vi "2 Cube Auto.vi"(11 "Right?":bool=TRUE) -> ()   [LabVIEW 2017]
uses:
  2 Cube Auto Type Def.ctl
  LabVIEW_is_Under_Control.lib/Util/Unpack Gamepad/D-Pad.ctl
  LabVIEW_is_Under_Control.lib/Util/Unpack Gamepad/Button Cluster.ctl
  Team Code/Robot Global Data.vi
panel:
  out "Enum":T1=enum."Finalizando"
  in  "Time to wait 4 (min 50ms)":dbl=50.0
  in  "DistanceFwd 4":dbl=100.0
  in  "Delay Fwd 4":i32=600
  in  "Time_Limit_fwd 4":dbl=2000.0 format="%#_13g"
  in  "Time_Limit_Turn 2":dbl=2000.0 format="%#_13g"
  in  "Turn 2":dbl=-110.0 format="%#_13g"
  in  "Delay Turn 2":i32=300
  in  "DistanceFwd 3":dbl=-60.0
  in  "Delay Fwd 3":i32=80
  in  "Time_Limit_fwd 3":dbl=2000.0 format="%#_13g"
  in  "Time to wait 3 (min 50ms)":dbl=50.0
  in  "DistanceFwd 2":dbl=55.0
  in  "Delay Fwd 2":i32=80
  in  "Time_Limit_fwd 2":dbl=1000.0 format="%#_13g"
  in  "Time to wait 2 (min 50ms)":dbl=50.0
  in  "Time_Limit_Turn":dbl=1500.0 format="%#_13g"
  in  "Turn":dbl=-30.0 format="%#_13g"
  in  "Delay Turn":i32=100
  in  "DistanceFwd":dbl=600.0
  in  "Delay Fwd":i32=300
  in  "Time_Limit_fwd":dbl=4800.0 format="%#_13g"
  in  "Time to wait (min 50ms)":dbl=100.0
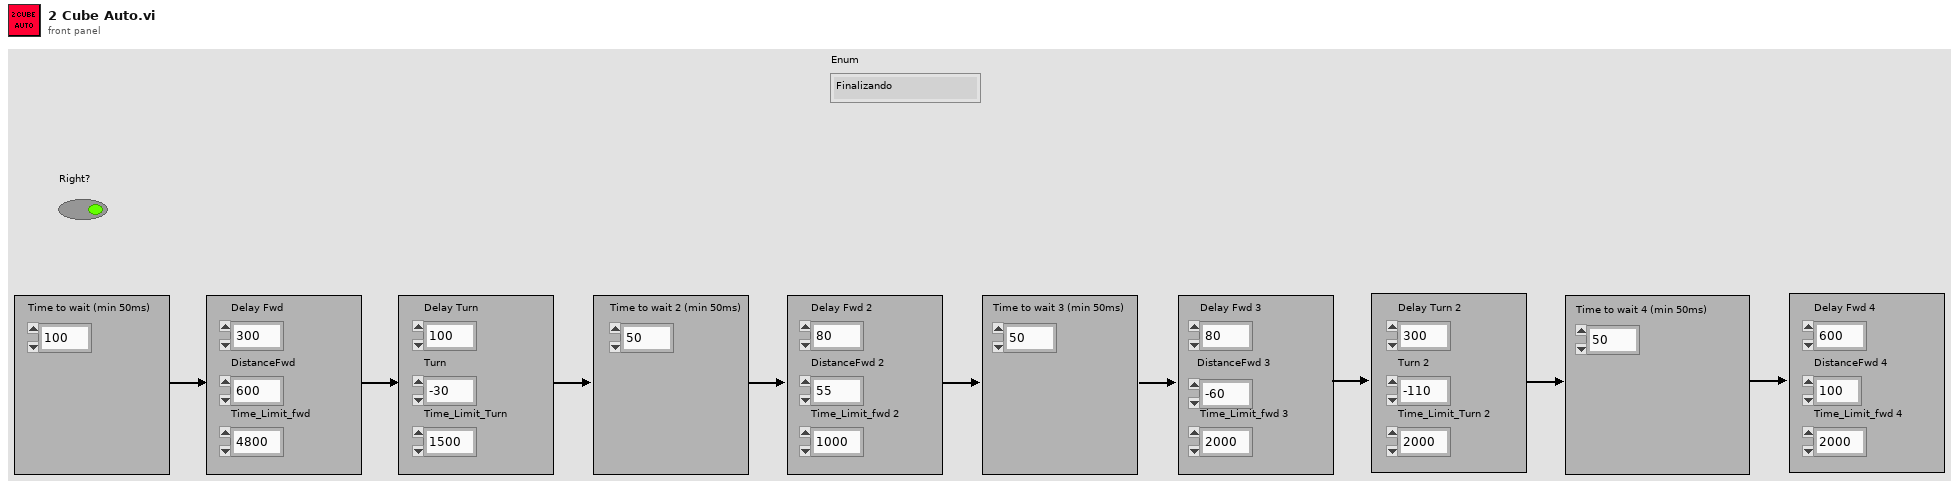
[diagram p1: front panel]
types:
  T1 = typedef "2 Cube Auto Type Def.ctl" = enum16{"Zerandosensor", "Andando", "Girando", "Zerandosensor2", "Andando2", "Score", "Zerandosensor3", "Andando3", "Girando2", "Zerandosensor4", "Andando4", "Elevator Up", "Score2", "Finalizando"}
  T2 = typedef "D-Pad.ctl" = cluster{"Top":bool, "Bottom":bool, "None":bool, "Right":bool, "Left":bool}
  T3 = cluster{"proportional gain (Kc)":dbl, "integral time (Ti, min)":dbl, "derivative time (Td, min)":dbl}
  T4 = typedef "Button Cluster.ctl" = cluster{"Buttons[0]":bool, "Buttons[1]":bool, "Buttons[2]":bool, "Buttons[3]":bool, "Buttons[4]":bool, "Buttons[5]":bool, "Buttons[6]":bool, "Buttons[7]":bool, "Buttons[8]":bool, "Buttons[9]":bool}
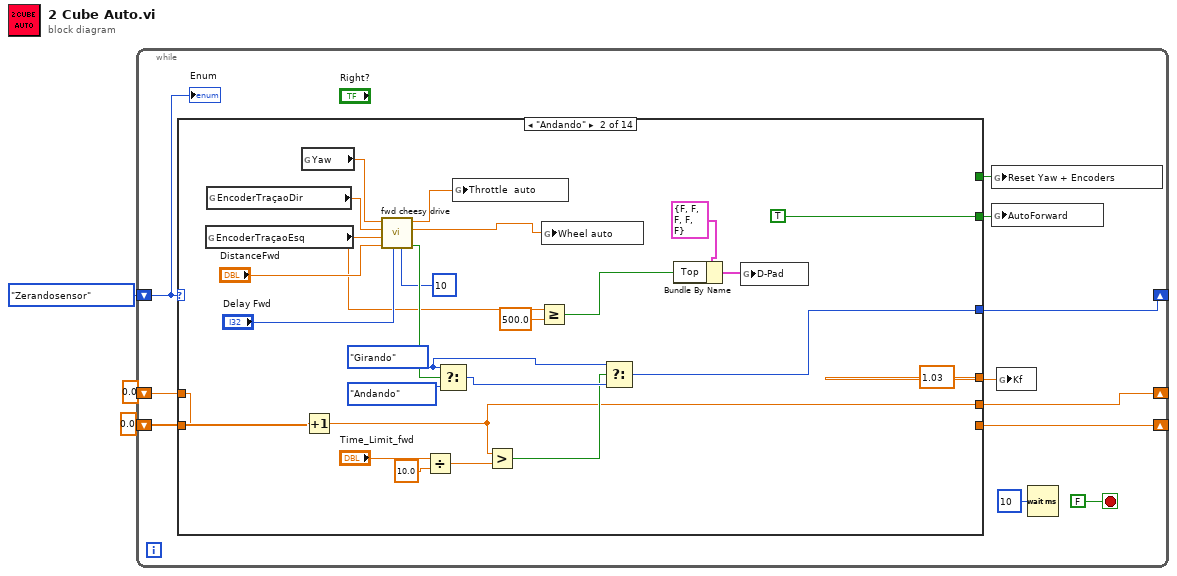
[diagram p0: block diagram]
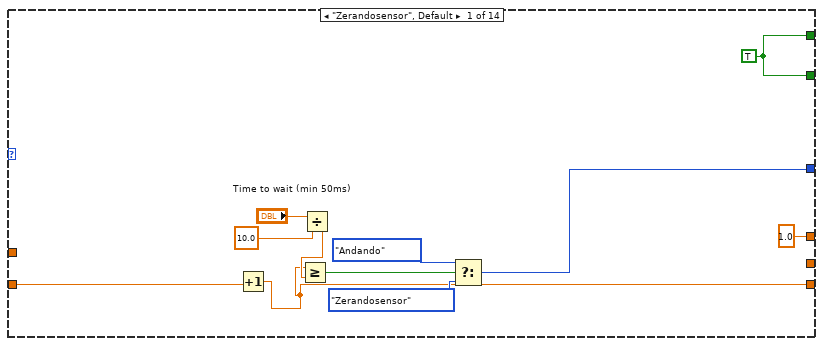
[diagram p2: hidden frame]
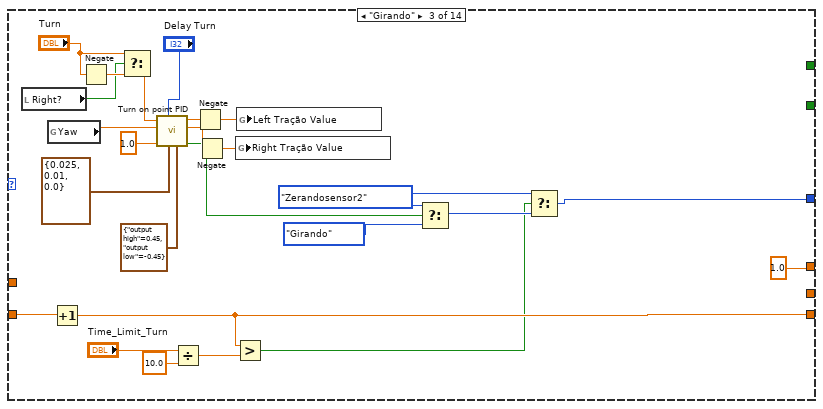
[diagram p3: hidden frame]
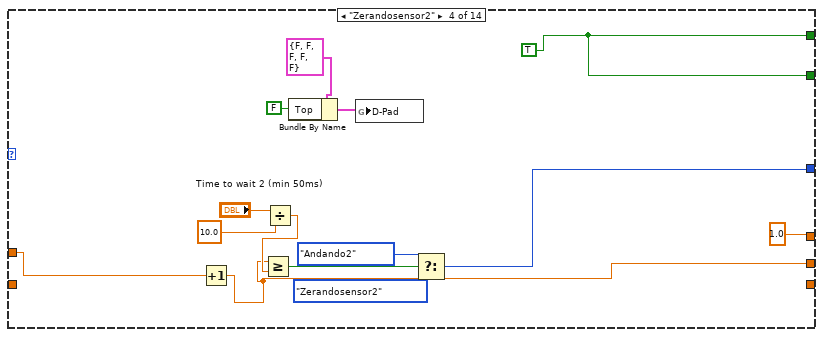
[diagram p4: hidden frame]
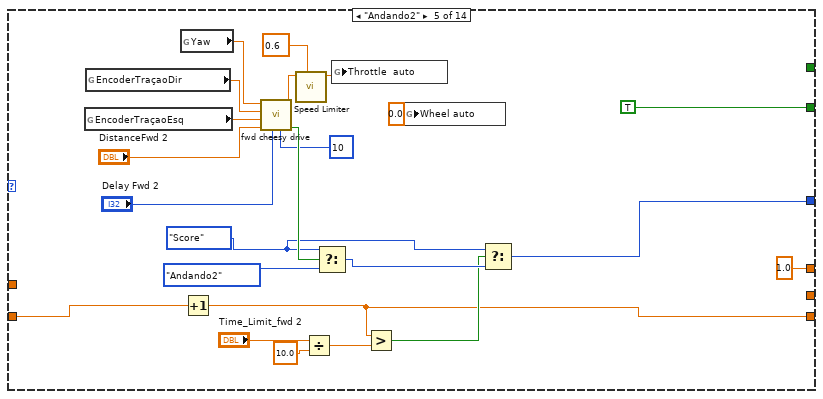
[diagram p5: hidden frame]
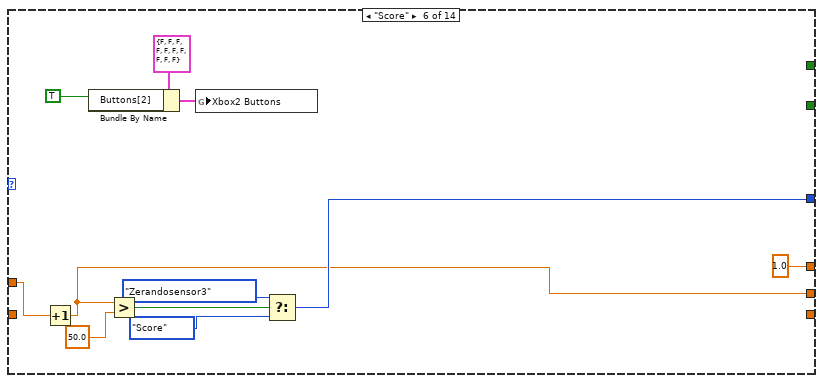
[diagram p6: hidden frame]
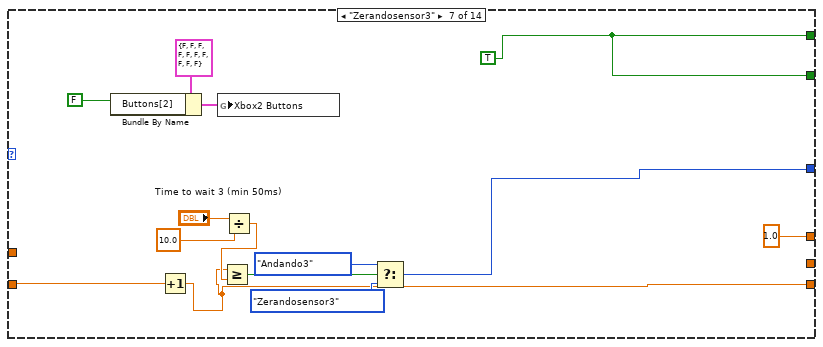
[diagram p7: hidden frame]
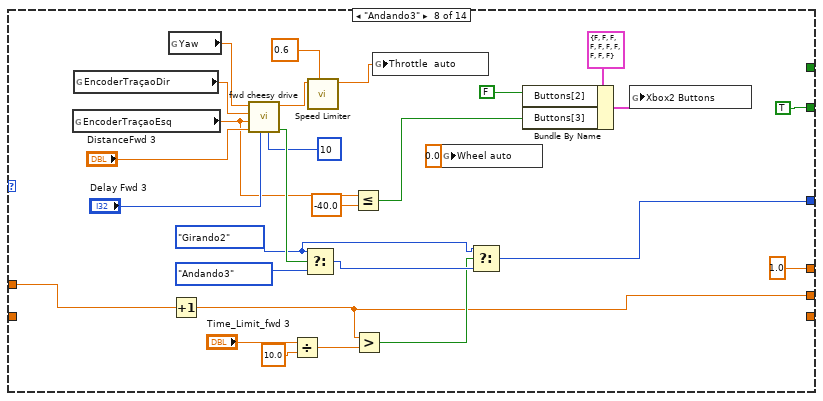
[diagram p8: hidden frame]
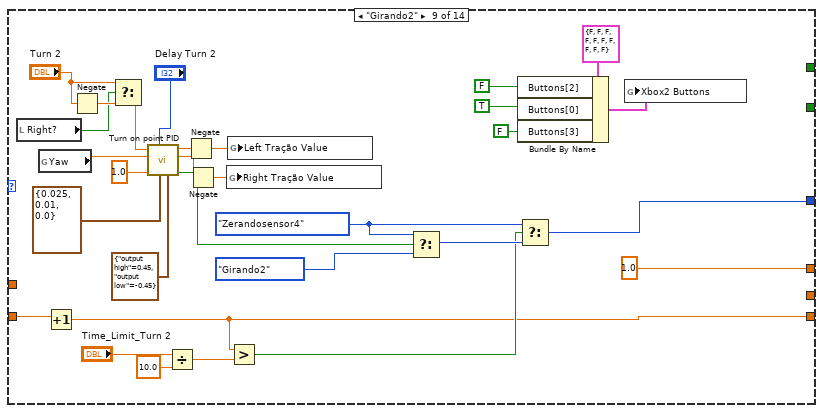
[diagram p9: hidden frame]
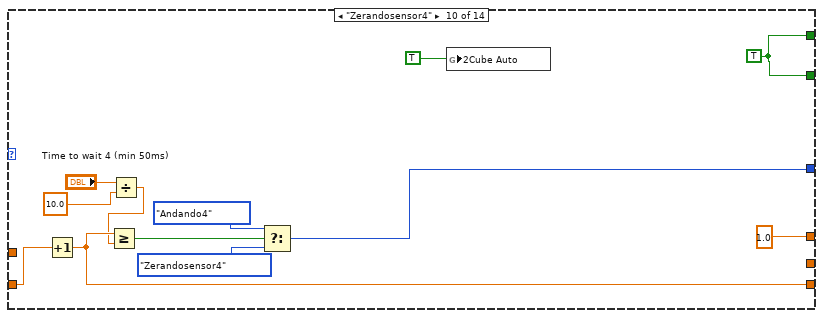
[diagram p10: hidden frame]
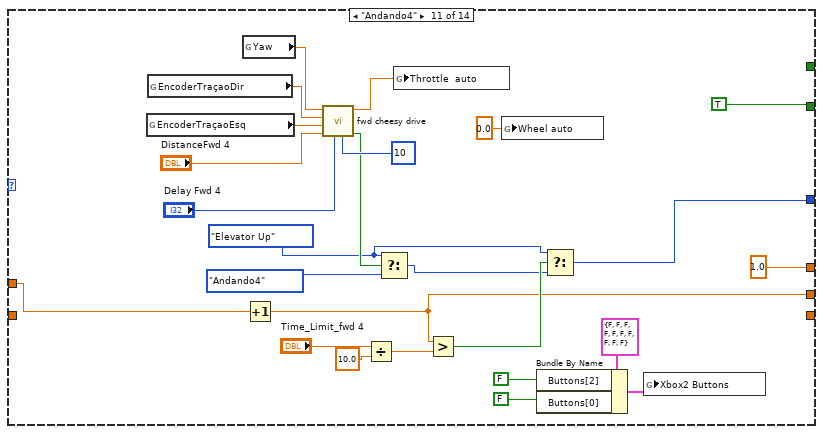
[diagram p11: hidden frame]
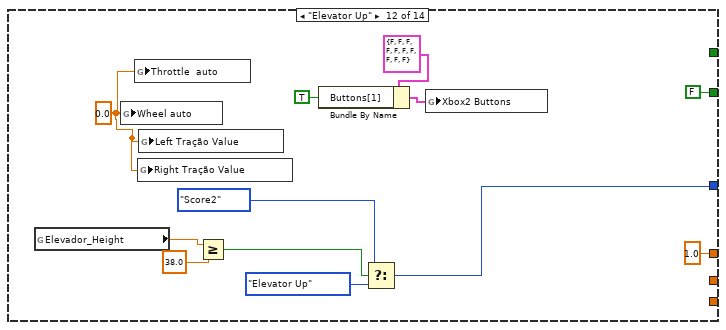
[diagram p12: hidden frame]
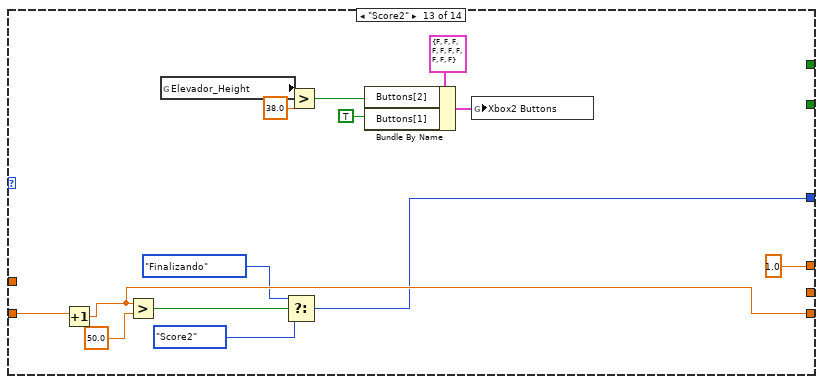
[diagram p13: hidden frame]
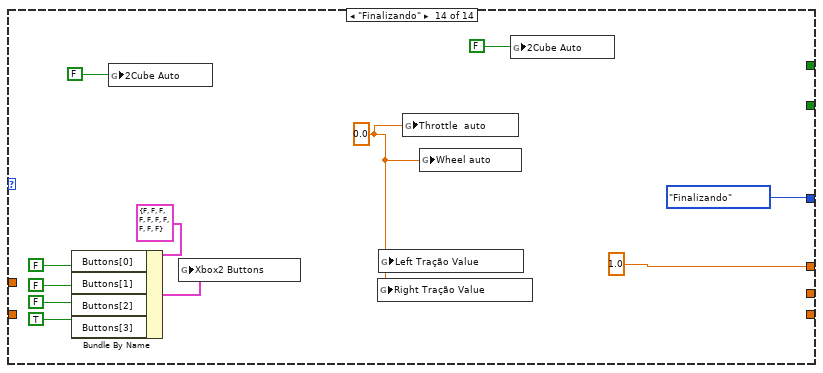
[diagram p14: hidden frame]
diagram:
  (unwired) 0.0
  n1 = while {
    shift-right: [w9] -> _
    shift-left: 2_Cube_Auto_Type_Def."Zerandosensor" ("Enum") -> [w3]
    shift-right: [w10] -> _
    shift-left: 0.0 -> [w11]
    shift-right: [w5] -> _
    shift-left: _ -> [w6]
    stop <- FALSE stop-if-true
    n2 = case shown="\"Andando\"" w3 {
      tunnel: w11 -> [w21 _ w71 _ w99 _ w131 _ w173 w197 _ _ w252 _]
      tunnel: [w14 _ w70 _ w98 _ w123 _ w172 w196 _ _ w251 _] -> w10
      tunnel: [w20 w43 w57 w84 w97 w117 w132 w151 w178 w199 w212 w234 w248 2_Cube_Auto_Type_Def."Finalizando" ("Enum")] -> w9
      tunnel: [w19 _ _ w83 _ _ w133 _ _ w201 _ _ _ _] -> w8
      tunnel: [w19 TRUE _ w83 TRUE _ w133 TRUE _ w201 TRUE FALSE _ _] -> w7
      tunnel: w6 -> [_ w36 _ w85 _ w116 _ w153 _ _ w217 _ _ _]
      tunnel: [_ w35 _ w75 _ w115 _ w152 _ _ w216 _ _ _] -> w5
      tunnel: [1.0 1.03 1.0 1.0 1.0 1.0 1.0 1.0 1.0 1.0 1.0 1.0 1.0 1.0] -> w4
      frame "Zerandosensor", Default {
        w19 = TRUE
        n3 = Increment(x=w21) -> (x+1=w14:dbl)
        n4 = Divide(x="Time to wait (min 50ms)", y=10.0) -> (x/y=w15:dbl)
        n5 = Greater Or Equal?(x=w14, y=w15) -> (x >= y?=w22:bool)
        n6 = Select(t=2_Cube_Auto_Type_Def."Andando" ("Enum"), s=w22, f=2_Cube_Auto_Type_Def."Zerandosensor" ("Enum")) -> (s? t:f=w20:T1)
      }
      frame "Andando" {
        w28 = 2_Cube_Auto_Type_Def."Girando" ("Enum")
        n7 = global read "Robot Global Data.vi" "EncoderTraçaoEsq"() -> (w26:dbl)
        n8 = global read "Robot Global Data.vi" "EncoderTraçaoDir"() -> (w48:dbl)
        n9 = global read "Robot Global Data.vi" "Yaw"() -> (w49:dbl)
        n10 = Increment(x=w36) -> (x+1=w35:dbl)
        n11 = call "fwd cheesy drive.vi"("Loop Timer"=10, "Time to stop"="Delay Fwd", "Distance"="DistanceFwd", "Encoder Left"=w26, "Encoder Right"=w48, "Yaw"=w49) -> ("Finished distance"=w37:bool, "Direction"=w25:dbl, "Trottle"=w46:dbl)  [unwired: 2 in, 1 out]
        n12 = Divide(x="Time_Limit_fwd", y=10.0) -> (x/y=w42:dbl)
        n13 = Select(t=w28, s=w37, f=2_Cube_Auto_Type_Def."Andando" ("Enum")) -> (s? t:f=w44:T1)
        n14 = global write "Robot Global Data.vi" "Throttle  auto"(w46) -> ()
        n15 = Greater?(x=w35, y=w42) -> (0:w39:bool)
        n16 = Greater Or Equal?(x=w26, y=500.0) -> (x >= y?=w31:bool)
        n17 = global write "Robot Global Data.vi" "Wheel auto"(w25) -> ()
        n18 = Select(t=w28, s=w39, f=w44) -> (s? t:f=w43:T1)
        n19 = Bundle By Name(cluster=T2 {"Top"=FALSE, "Bottom"=FALSE, "None"=FALSE, "Right"=FALSE, "Left"=FALSE} ("D-Pad"), "Top"=w31) -> (w33:T2)
        n20 = global write "Robot Global Data.vi" "D-Pad"(w33) -> ()
      }
      frame "Girando" {
        w53 = 2_Cube_Auto_Type_Def."Zerandosensor2" ("Enum")
        n21 = local read "Right?"() -> (w50:bool)
        n22 = global read "Robot Global Data.vi" "Yaw"() -> (w66:dbl)
        n23 = Increment(x=w71) -> (x+1=w70:dbl)
        n24 = Negate(x="Turn") -> (-x=w56:dbl)
        n25 = Select(t="Turn", s=w50, f=w56) -> (s? t:f=w54:dbl)
        n26 = call "Turn on point PID.vi"("Range"=cluster{"output high":dbl, "output low":dbl} {"output high"=0.45, "output low"=-0.45}, "Gains"=T3 {"proportional gain (Kc)"=0.025, "integral time (Ti, min)"=0.01, "derivative time (Td, min)"=0.0}, "Time to stop"="Delay Turn", "Precision"=1.0, "Yaw"=w66, "Setpoint(degrees)"=w54) -> ("Finished?"=w62:bool, "PWM right"=w65:dbl, "PWM left"=w64:dbl)  [unwired: 3 in]
        n27 = Divide(x="Time_Limit_Turn", y=10.0) -> (x/y=w73:dbl)
        n28 = Negate(x=w64) -> (-x=w67:dbl)
        n29 = Negate(x=w65) -> (-x=w68:dbl)
        n30 = Greater?(x=w70, y=w73) -> (0:w58:bool)
        n31 = global write "Robot Global Data.vi" "Right Tração Value"(w68) -> ()
        n32 = global write "Robot Global Data.vi" "Left Tração Value"(w67) -> ()
        n33 = Select(t=w53, s=w62, f=2_Cube_Auto_Type_Def."Girando" ("Enum")) -> (s? t:f=w69:T1)
        n34 = Select(t=w53, s=w58, f=w69) -> (s? t:f=w57:T1)
      }
      frame "Zerandosensor2" {
        w83 = TRUE
        n35 = Increment(x=w85) -> (x+1=w75:dbl)
        n36 = Divide(x="Time to wait 2 (min 50ms)", y=10.0) -> (x/y=w76:dbl)
        n37 = Greater Or Equal?(x=w75, y=w76) -> (x >= y?=w86:bool)
        n38 = Bundle By Name(cluster=T2 {"Top"=FALSE, "Bottom"=FALSE, "None"=FALSE, "Right"=FALSE, "Left"=FALSE} ("D-Pad"), "Top"=FALSE) -> (w82:T2)
        n39 = global write "Robot Global Data.vi" "D-Pad"(w82) -> ()
        n40 = Select(t=2_Cube_Auto_Type_Def."Andando2" ("Enum"), s=w86, f=2_Cube_Auto_Type_Def."Zerandosensor2" ("Enum")) -> (s? t:f=w84:T1)
      }
      frame "Andando2" {
        w90 = 2_Cube_Auto_Type_Def."Score" ("Enum")
        n41 = global read "Robot Global Data.vi" "EncoderTraçaoEsq"() -> (w110:dbl)
        n42 = global read "Robot Global Data.vi" "EncoderTraçaoDir"() -> (w109:dbl)
        n43 = global read "Robot Global Data.vi" "Yaw"() -> (w111:dbl)
        n44 = Increment(x=w99) -> (x+1=w98:dbl)
        n45 = call "fwd cheesy drive.vi"("Loop Timer"=10, "Time to stop"="Delay Fwd 2", "Distance"="DistanceFwd 2", "Encoder Left"=w110, "Encoder Right"=w109, "Yaw"=w111) -> ("Finished distance"=w101:bool, "Trottle"=w93:dbl)  [unwired: 2 in, 2 out]
        n46 = call "Speed Limiter.vi"("Limit"=0.6, "Motor Input"=w93) -> ("Output"=w94:dbl)  [unwired: 9 in]
        n47 = Divide(x="Time_Limit_fwd 2", y=10.0) -> (x/y=w105:dbl)
        n48 = Select(t=w90, s=w101, f=2_Cube_Auto_Type_Def."Andando2" ("Enum")) -> (s? t:f=w106:T1)
        n49 = global write "Robot Global Data.vi" "Throttle  auto"(w94) -> ()
        n50 = Greater?(x=w98, y=w105) -> (0:w102:bool)
        n51 = global write "Robot Global Data.vi" "Wheel auto"(0.0 ("Wheel auto")) -> ()
        n52 = Select(t=w90, s=w102, f=w106) -> (s? t:f=w97:T1)
      }
      frame "Score" {
        n53 = Increment(x=w116) -> (x+1=w115:dbl)
        n54 = Bundle By Name(cluster=T4 {"Buttons[0]"=FALSE, "Buttons[1]"=FALSE, "Buttons[2]"=FALSE, "Buttons[3]"=FALSE, "Buttons[4]"=FALSE, "Buttons[5]"=FALSE, "Buttons[6]"=FALSE, "Buttons[7]"=FALSE, "Buttons[8]"=FALSE, "Buttons[9]"=FALSE} ("Xbox Buttons"), "Buttons[2]"=TRUE) -> (w121:T4)
        n55 = Greater?(x=w115, y=50.0) -> (0:w118:bool)
        n56 = global write "Robot Global Data.vi" "Xbox2 Buttons"(w121) -> ()
        n57 = Select(t=2_Cube_Auto_Type_Def."Zerandosensor3" ("Enum"), s=w118, f=2_Cube_Auto_Type_Def."Score" ("Enum")) -> (s? t:f=w117:T1)
      }
      frame "Zerandosensor3" {
        w133 = TRUE
        n58 = Bundle By Name(cluster=T4 {"Buttons[0]"=FALSE, "Buttons[1]"=FALSE, "Buttons[2]"=FALSE, "Buttons[3]"=FALSE, "Buttons[4]"=FALSE, "Buttons[5]"=FALSE, "Buttons[6]"=FALSE, "Buttons[7]"=FALSE, "Buttons[8]"=FALSE, "Buttons[9]"=FALSE} ("Xbox Buttons"), "Buttons[2]"=FALSE) -> (w126:T4)
        n59 = Increment(x=w131) -> (x+1=w123:dbl)
        n60 = global write "Robot Global Data.vi" "Xbox2 Buttons"(w126) -> ()
        n61 = Divide(x="Time to wait 3 (min 50ms)", y=10.0) -> (x/y=w124:dbl)
        n62 = Greater Or Equal?(x=w123, y=w124) -> (x >= y?=w134:bool)
        n63 = Select(t=2_Cube_Auto_Type_Def."Andando3" ("Enum"), s=w134, f=2_Cube_Auto_Type_Def."Zerandosensor3" ("Enum")) -> (s? t:f=w132:T1)
      }
      frame "Andando3" {
        w147 = 2_Cube_Auto_Type_Def."Girando2" ("Enum")
        n64 = global read "Robot Global Data.vi" "EncoderTraçaoEsq"() -> (w139:dbl)
        n65 = global read "Robot Global Data.vi" "EncoderTraçaoDir"() -> (w163:dbl)
        n66 = global read "Robot Global Data.vi" "Yaw"() -> (w164:dbl)
        n67 = Increment(x=w153) -> (x+1=w152:dbl)
        n68 = call "fwd cheesy drive.vi"("Loop Timer"=10, "Time to stop"="Delay Fwd 3", "Distance"="DistanceFwd 3", "Encoder Left"=w139, "Encoder Right"=w163, "Yaw"=w164) -> ("Finished distance"=w155:bool, "Trottle"=w142:dbl)  [unwired: 2 in, 2 out]
        n69 = Divide(x="Time_Limit_fwd 3", y=10.0) -> (x/y=w159:dbl)
        n70 = Select(t=w147, s=w155, f=2_Cube_Auto_Type_Def."Andando3" ("Enum")) -> (s? t:f=w160:T1)
        n71 = call "Speed Limiter.vi"("Limit"=0.6, "Motor Input"=w142) -> ("Output"=w141:dbl)  [unwired: 9 in]
        n72 = Less Or Equal?(x=w139, y=-40.0) -> (x <= y?=w137:bool)
        n73 = Greater?(x=w152, y=w159) -> (0:w156:bool)
        n74 = global write "Robot Global Data.vi" "Throttle  auto"(w141) -> ()
        n75 = global write "Robot Global Data.vi" "Wheel auto"(0.0 ("Wheel auto")) -> ()
        n76 = Select(t=w147, s=w156, f=w160) -> (s? t:f=w151:T1)
        n77 = Bundle By Name(cluster=T4 {"Buttons[0]"=FALSE, "Buttons[1]"=FALSE, "Buttons[2]"=FALSE, "Buttons[3]"=FALSE, "Buttons[4]"=FALSE, "Buttons[5]"=FALSE, "Buttons[6]"=FALSE, "Buttons[7]"=FALSE, "Buttons[8]"=FALSE, "Buttons[9]"=FALSE} ("Xbox Buttons"), "Buttons[2]"=FALSE, "Buttons[3]"=w137) -> (w144:T4)
        n78 = global write "Robot Global Data.vi" "Xbox2 Buttons"(w144) -> ()
      }
      frame "Girando2" {
        w180 = 2_Cube_Auto_Type_Def."Zerandosensor4" ("Enum")
        n79 = local read "Right?"() -> (w170:bool)
        n80 = global read "Robot Global Data.vi" "Yaw"() -> (w184:dbl)
        n81 = Increment(x=w173) -> (x+1=w172:dbl)
        n82 = Negate(x="Turn 2") -> (-x=w192:dbl)
        n83 = Select(t="Turn 2", s=w170, f=w192) -> (s? t:f=w194:dbl)
        n84 = call "Turn on point PID.vi"("Range"=cluster{"output high":dbl, "output low":dbl} {"output high"=0.45, "output low"=-0.45}, "Gains"=T3 {"proportional gain (Kc)"=0.025, "integral time (Ti, min)"=0.01, "derivative time (Td, min)"=0.0}, "Time to stop"="Delay Turn 2", "Precision"=1.0, "Yaw"=w184, "Setpoint(degrees)"=w194) -> ("Finished?"=w188:bool, "PWM right"=w185:dbl, "PWM left"=w186:dbl)  [unwired: 3 in]
        n85 = Divide(x="Time_Limit_Turn 2", y=10.0) -> (x/y=w176:dbl)
        n86 = Negate(x=w186) -> (-x=w183:dbl)
        n87 = Negate(x=w185) -> (-x=w182:dbl)
        n88 = global write "Robot Global Data.vi" "Right Tração Value"(w182) -> ()
        n89 = global write "Robot Global Data.vi" "Left Tração Value"(w183) -> ()
        n90 = Greater?(x=w172, y=w176) -> (0:w174:bool)
        n91 = Select(t=w180, s=w188, f=2_Cube_Auto_Type_Def."Girando2" ("Enum")) -> (s? t:f=w181:T1)
        n92 = Bundle By Name(cluster=T4 {"Buttons[0]"=FALSE, "Buttons[1]"=FALSE, "Buttons[2]"=FALSE, "Buttons[3]"=FALSE, "Buttons[4]"=FALSE, "Buttons[5]"=FALSE, "Buttons[6]"=FALSE, "Buttons[7]"=FALSE, "Buttons[8]"=FALSE, "Buttons[9]"=FALSE} ("Xbox Buttons"), "Buttons[2]"=FALSE, "Buttons[0]"=TRUE ("Buttons[1]"), "Buttons[3]"=FALSE) -> (w168:T4)
        n93 = Select(t=w180, s=w174, f=w181) -> (s? t:f=w178:T1)
        n94 = global write "Robot Global Data.vi" "Xbox2 Buttons"(w168) -> ()
      }
      frame "Zerandosensor4" {
        w201 = TRUE
        n95 = Increment(x=w197) -> (x+1=w196:dbl)
        n96 = Divide(x="Time to wait 4 (min 50ms)", y=10.0) -> (x/y=w195:dbl)
        n97 = Greater Or Equal?(x=w196, y=w195) -> (x >= y?=w205:bool)
        n98 = Select(t=2_Cube_Auto_Type_Def."Andando4" ("Enum"), s=w205, f=2_Cube_Auto_Type_Def."Zerandosensor4" ("Enum")) -> (s? t:f=w199:T1)
        n99 = global write "Robot Global Data.vi" "2Cube Auto"(TRUE) -> ()
      }
      frame "Andando4" {
        w213 = 2_Cube_Auto_Type_Def."Elevator Up" ("Enum")
        n100 = global read "Robot Global Data.vi" "EncoderTraçaoEsq"() -> (w231:dbl)
        n101 = global read "Robot Global Data.vi" "EncoderTraçaoDir"() -> (w220:dbl)
        n102 = global read "Robot Global Data.vi" "Yaw"() -> (w219:dbl)
        n103 = Increment(x=w217) -> (x+1=w216:dbl)
        n104 = call "fwd cheesy drive.vi"("Loop Timer"=10, "Time to stop"="Delay Fwd 4", "Distance"="DistanceFwd 4", "Encoder Left"=w231, "Encoder Right"=w220, "Yaw"=w219) -> ("Finished distance"=w229:bool, "Trottle"=w222:dbl)  [unwired: 2 in, 2 out]
        n105 = Divide(x="Time_Limit_fwd 4", y=10.0) -> (x/y=w225:dbl)
        n106 = Select(t=w213, s=w229, f=2_Cube_Auto_Type_Def."Andando4" ("Enum")) -> (s? t:f=w224:T1)
        n107 = global write "Robot Global Data.vi" "Throttle  auto"(w222) -> ()
        n108 = Greater?(x=w216, y=w225) -> (0:w228:bool)
        n109 = global write "Robot Global Data.vi" "Wheel auto"(0.0 ("Wheel auto")) -> ()
        n110 = Bundle By Name(cluster=T4 {"Buttons[0]"=FALSE, "Buttons[1]"=FALSE, "Buttons[2]"=FALSE, "Buttons[3]"=FALSE, "Buttons[4]"=FALSE, "Buttons[5]"=FALSE, "Buttons[6]"=FALSE, "Buttons[7]"=FALSE, "Buttons[8]"=FALSE, "Buttons[9]"=FALSE} ("Xbox Buttons"), "Buttons[2]"=FALSE, "Buttons[0]"=FALSE ("Buttons[1]")) -> (w210:T4)
        n111 = Select(t=w213, s=w228, f=w224) -> (s? t:f=w212:T1)
        n112 = global write "Robot Global Data.vi" "Xbox2 Buttons"(w210) -> ()
      }
      frame "Elevator Up" {
        w232 = 0.0 ("Wheel auto")
        n113 = global read "Robot Global Data.vi" "Elevador_Height"() -> (w239:dbl)
        n114 = global write "Robot Global Data.vi" "Wheel auto"(w232) -> ()
        n115 = global write "Robot Global Data.vi" "Throttle  auto"(w232) -> ()
        n116 = global write "Robot Global Data.vi" "Right Tração Value"(w232) -> ()
        n117 = global write "Robot Global Data.vi" "Left Tração Value"(w232) -> ()
        n118 = Greater Or Equal?(x=w239, y=38.0) -> (x >= y?=w237:bool)
        n119 = Bundle By Name(cluster=T4 {"Buttons[0]"=FALSE, "Buttons[1]"=FALSE, "Buttons[2]"=FALSE, "Buttons[3]"=FALSE, "Buttons[4]"=FALSE, "Buttons[5]"=FALSE, "Buttons[6]"=FALSE, "Buttons[7]"=FALSE, "Buttons[8]"=FALSE, "Buttons[9]"=FALSE} ("Xbox Buttons"), "Buttons[1]"=TRUE) -> (w241:T4)
        n120 = Select(t=2_Cube_Auto_Type_Def."Score2" ("Enum"), s=w237, f=2_Cube_Auto_Type_Def."Elevator Up") -> (s? t:f=w234:T1)
        n121 = global write "Robot Global Data.vi" "Xbox2 Buttons"(w241) -> ()
      }
      frame "Score2" {
        n122 = Increment(x=w252) -> (x+1=w251:dbl)
        n123 = Greater?(x=w251, y=50.0) -> (0:w254:bool)
        n124 = global read "Robot Global Data.vi" "Elevador_Height"() -> (w246:dbl)
        n125 = Select(t=2_Cube_Auto_Type_Def."Finalizando" ("Enum"), s=w254, f=2_Cube_Auto_Type_Def."Score2" ("Enum")) -> (s? t:f=w248:T1)
        n126 = Greater?(x=w246, y=38.0) -> (0:w244:bool)
        n127 = Bundle By Name(cluster=T4 {"Buttons[0]"=FALSE, "Buttons[1]"=FALSE, "Buttons[2]"=FALSE, "Buttons[3]"=FALSE, "Buttons[4]"=FALSE, "Buttons[5]"=FALSE, "Buttons[6]"=FALSE, "Buttons[7]"=FALSE, "Buttons[8]"=FALSE, "Buttons[9]"=FALSE} ("Xbox Buttons"), "Buttons[2]"=w244, "Buttons[1]"=TRUE) -> (w257:T4)
        n128 = global write "Robot Global Data.vi" "Xbox2 Buttons"(w257) -> ()
      }
      frame "Finalizando" {
        w267 = 0.0
        n129 = Bundle By Name(cluster=T4 {"Buttons[0]"=FALSE, "Buttons[1]"=FALSE, "Buttons[2]"=FALSE, "Buttons[3]"=FALSE, "Buttons[4]"=FALSE, "Buttons[5]"=FALSE, "Buttons[6]"=FALSE, "Buttons[7]"=FALSE, "Buttons[8]"=FALSE, "Buttons[9]"=FALSE} ("Xbox Buttons"), "Buttons[0]"=FALSE ("Buttons[2]"), "Buttons[1]"=FALSE ("Buttons[3]"), "Buttons[2]"=FALSE ("Buttons[1]"), "Buttons[3]"=TRUE ("Buttons[0]")) -> (w268:T4)
        n130 = global write "Robot Global Data.vi" "2Cube Auto"(FALSE) -> ()
        n131 = global write "Robot Global Data.vi" "Xbox2 Buttons"(w268) -> ()
        n132 = global write "Robot Global Data.vi" "Right Tração Value"(w267) -> ()
        n133 = global write "Robot Global Data.vi" "Left Tração Value"(w267) -> ()
        n134 = global write "Robot Global Data.vi" "Throttle  auto"(w267) -> ()
        n135 = global write "Robot Global Data.vi" "Wheel auto"(w267) -> ()
        n136 = global write "Robot Global Data.vi" "2Cube Auto"(FALSE) -> ()
      }
    }
    n137 = global write "Robot Global Data.vi" "Reset Yaw + Encoders"(w8) -> ()
    n138 = global write "Robot Global Data.vi" "AutoForward"(w7) -> ()
    n139 = global write "Robot Global Data.vi" "Kf"(w4) -> ()
    n140 = Wait (ms)(milliseconds to wait=u32 10) -> ()  [unwired: 1 out]
    "Enum" <- w3
  }
